vi "Export Asset Configuration.vi"(8 "error in (no error)":errorcluster, 9 "Ouput Directory":path, 11 "InsightCM Console Wrapper in":refnum<class "InsightCM Console Wrapper.lvclass">) -> (0 "error out":errorcluster, 3 "InsightCM Console Wrapper out":refnum<class "InsightCM Console Wrapper.lvclass">)   [LabVIEW 2020, in "InsightCM Console Wrapper.lvclass"]
doc: "Export asset configuration as an Excel File.\n\nConsole command -> exportassetspreadsheet -o [output filepath]"
uses:
  InsightCM Console Wrapper.lvclass
  C:/Users/fflores/Documents/GitHub Projects/LabVIEW-CLI-Wrapper/Console Wrapper/Console Wrapper.lvclass
  Console Wrapper/Console Wrapper.lvclass/Console Wrapper.ctl
  Console Wrapper/Write Command Options.vi
  Console Wrapper/Write Command.vi
  Console Wrapper/Console Wrapper.lvclass
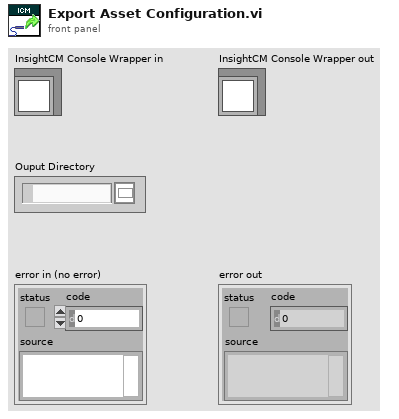
[diagram p1: front panel]
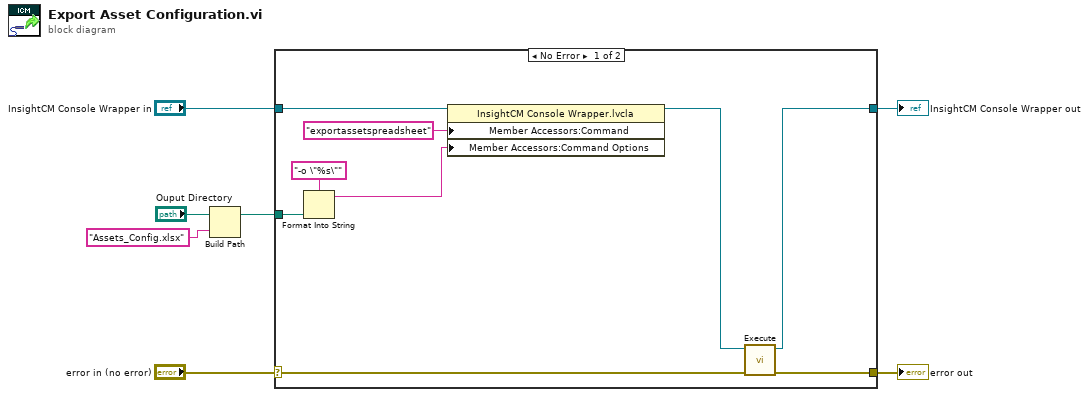
[diagram p0: block diagram]
diagram:
  n1 = Build Path(base path="Ouput Directory", name or relative path="Assets_Config.xlsx") -> (appended path=w2:path)
  n2 = case shown="No Error" "error in (no error)" {
    selector: "error in (no error)" -> [w16 w18]
    tunnel: [w15 w18] -> w6
    tunnel: [w13 w17] -> w4
    tunnel: "InsightCM Console Wrapper in" -> [w14 w17]
    tunnel: w2 -> [w9 _]
    frame No Error {
      n3 = Format Into String(format string="-o \"%s\"", w9) -> (resulting string=w10:string)  [unwired: 2 in, 1 out]
      n4 = property class="InsightCM Console Wrapper.lvcla"(reference=w14, "Member Accessors:Command"="exportassetspreadsheet" ("Command"), "Member Accessors:Command Options"=w10) -> (reference out=w12:refnum<class "InsightCM Console Wrapper.lvclass">)  [unwired: 1 in, 1 out]
      n5 = call "Execute.vi"("error in (no error)"=w16, "Console Wrapper in"=w12) -> ("error out"=w15:errorcluster, "Console Wrapper out"=w13:refnum<class "InsightCM Console Wrapper.lvclass">)  [unwired: 7 in, 1 out]
    }
    frame Error {
    }
  }
  "error out" <- w6
  "InsightCM Console Wrapper out" <- w4
